vi "Test Process within Nested App Log When Logger Set for Intermediate App.vi"(8 "error in (no error)":errorcluster, 11 "Test Case In":refnum<class "Logger Test.lvclass">) -> (0 "error out":errorcluster, 3 "Test Case Out":refnum<class "Logger Test.lvclass">)   [LabVIEW 2020, in "Logger Test.lvclass"]
uses:
  Logger Test.lvclass
  Logger Test.lvclass/Logger Test.ctl
  source/Framework Test Suite/Mock Log Handler/Mock Log Handler.lvclass
  source/Framework/Process/Process.lvclass
  source/Framework/Application/Application.lvclass
  source/Framework Test Suite/Mock Process/Mock Process.lvclass
  source/Framework Test Suite/Support/Test Support.lvlib
  source/Framework/Logging/Logging.lvclass
  9c4a66fc-af29-4a58-8a71-606aefca4567.vi
  C:/Git/astemes-triarc-framework/source/Framework/Process/Process.lvclass
  C:/Git/astemes-triarc-framework/source/Framework/Base/Base.lvclass
  C:/Git/astemes-triarc-framework/source/Framework/Error Handler Interface/Error Handler Interface.lvclass
  C:/Git/astemes-triarc-framework/source/Framework/Logging/Logging.lvclass
  C:/Git/astemes-triarc-framework/source/Framework/Application/Application.lvclass
  C:/Git/astemes-triarc-framework/source/Framework/Async Handler/Async Handler.lvclass
  C:/Git/astemes-triarc-framework/source/Framework Test Suite/Mock Log Handler/Mock Log Handler.lvclass
  C:/Git/astemes-triarc-framework/source/Framework/Configuration File/Configuration File.lvclass
  C:/Git/astemes-triarc-framework/source/Framework/Configuration/Configuration.lvclass
  C:/Git/astemes-triarc-framework/source/Framework Test Suite/Mock Process/Mock Process.lvclass
  C:/Git/astemes-triarc-framework/source/Framework/Helper Loop/Helper Loop.lvclass
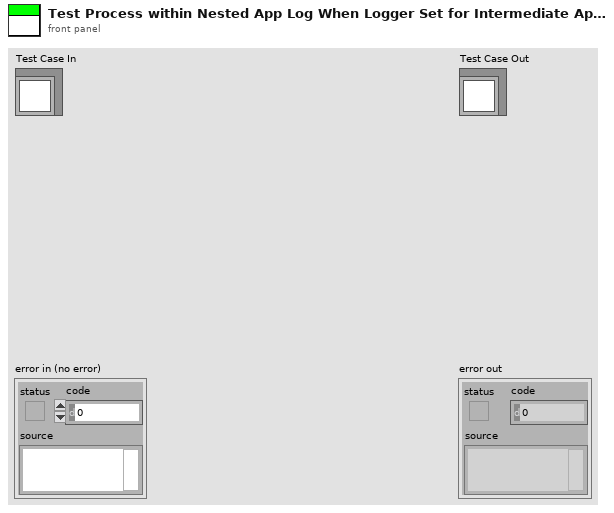
[diagram p1: front panel]
types:
  T1 = typedef "Mock Log Handler.lvclass/Log Entry.ctl" = cluster{"Level":string, "Source":string, "Message":string}
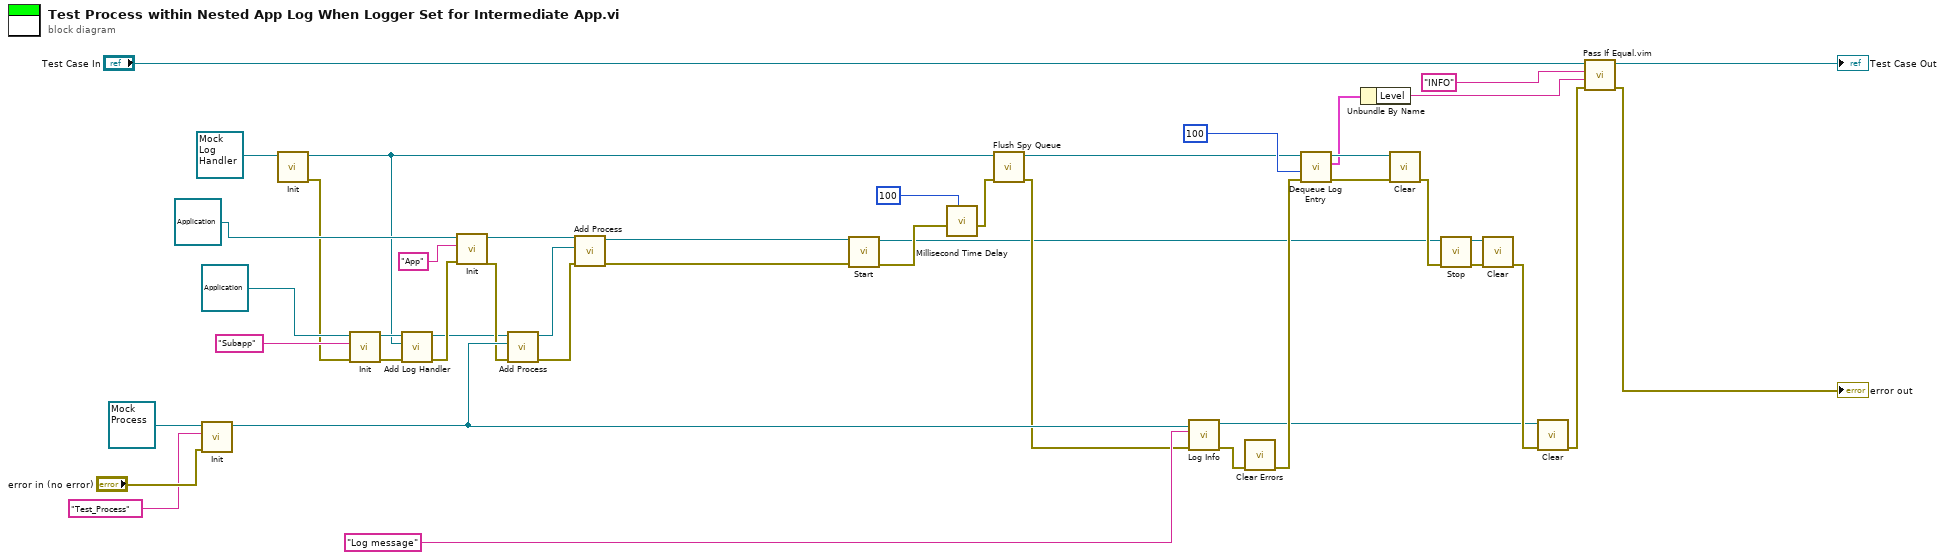
[diagram p0: block diagram]
diagram:
  n1 = call-dynamic "Init.vi"("error in (no error)"="error in (no error)", "Name"="Test_Process", "Mock Process In"=refnum<class "Mock Process.lvclass"> refnum) -> ("Mock Process Out"=w18:refnum<class "Mock Process.lvclass">)  [unwired: 7 in, 1 out]
  n2 = call-dynamic "Init.vi"("Mock Log Handler In"=refnum<class "Mock Log Handler.lvclass"> refnum ("Mock Log Handler.lvclass")) -> ("error out"=w6:errorcluster, "Mock Log Handler Out"=w1:refnum<class "Mock Log Handler.lvclass">)  [unwired: 9 in]
  n3 = call-dynamic "Init.vi"("error in (no error)"=w6, "Name"="Subapp", "Process In"=refnum<class "Application.lvclass"> refnum ("Application.lvclass")) -> ("error out"=w5:errorcluster, "Process Out"=w3:refnum<class "Application.lvclass">)  [unwired: 7 in]
  n4 = call "Add Log Handler.vi"("error in (no error)"=w5, "Log Handler"=w1, "Process In"=w3) -> ("error out"=w4:errorcluster, "Process Out"=w2:refnum<class "Application.lvclass">)  [unwired: 7 in]
  n5 = call-dynamic "Init.vi"("error in (no error)"=w4, "Name"="App", "Process In"=refnum<class "Application.lvclass"> refnum ("Application.lvclass")) -> ("error out"=w13:errorcluster, "Process Out"=w15:refnum<class "Application.lvclass">)  [unwired: 7 in]
  n6 = call "Add Process.vi"("error in (no error)"=w13, "Process"=w18, "Application In"=w2) -> ("error out"=w12:errorcluster, "Application Out"=w14:refnum<class "Application.lvclass">)  [unwired: 7 in]
  n7 = call "Add Process.vi"("error in (no error)"=w12, "Process"=w14, "Application In"=w15) -> ("error out"=w11:errorcluster, "Application Out"=w9:refnum<class "Application.lvclass">)  [unwired: 7 in]
  n8 = call "Start.vi"("error in (no error)"=w11, "Process In"=w9) -> ("error out"=w10:errorcluster, "Process Out"=w8:refnum<class "Application.lvclass">)  [unwired: 7 in, 1 out]
  n9 = call "Millisecond Time Delay.vi"("milliseconds to wait"=u32 100, "error in (no error)"=w10) -> ("error out"=w20:errorcluster)  [unwired: 7 in]
  n10 = call "Flush Spy Queue.vi"("error in (no error)"=w20, "Mock Log Handler in"=w1) -> ("error out"=w17:errorcluster, "Mock Log Handler out"=w21:refnum<class "Mock Log Handler.lvclass">)  [unwired: 7 in, 1 out]
  n11 = call "Log Info.vi"("error in (no error)"=w17, "Message"="Log message", "Logging In"=w18) -> ("error out"=w31:errorcluster, "Logging Out"=w22:refnum<class "Mock Process.lvclass">)  [unwired: 7 in]
  n12 = call <vilib>:"Clear Errors.vi"("error in (no error)"=w31) -> ("error out"=w30:errorcluster)  [unwired: 5 in, 1 out]
  n13 = call "Dequeue Log Entry.vi"("error in (no error)"=w30, "timeout in ms (-1)"=100, "Mock Log Handler in"=w21) -> ("error out"=w40:errorcluster, "Entry"=w37:T1, "Mock Log Handler out"=w41:refnum<class "Mock Log Handler.lvclass">)  [unwired: 5 in, 1 out]
  n14 = Unbundle By Name(w37) -> ("Level"=w36:string)
  n15 = call-dynamic "Clear.vi"("error in (no error)"=w40, "Mock Log Handler In"=w41) -> ("error out"=w38:errorcluster)  [unwired: 9 in]
  n16 = call "Stop.vi"("error in (no error)"=w38, "Process In"=w8) -> ("error out"=w24:errorcluster, "Process Out"=w23:refnum<class "Application.lvclass">)  [unwired: 7 in, 1 out]
  n17 = call-dynamic "Clear.vi"("error in (no error)"=w24, "Application In"=w23) -> ("error out"=w43:errorcluster)  [unwired: 9 in]
  n18 = call-dynamic "Clear.vi"("error in (no error)"=w43, "Mock Process In"=w22) -> ("error out"=w33:errorcluster)  [unwired: 9 in]
  n19 = call "Pass If Equal.vim"("error in (no error)"=w33, "Actual"=w36, "Expected"="INFO", "LUnit Test Case In"="Test Case In") -> ("error out"=→"error out":errorcluster, "LUnit Test Case Out"=→"Test Case Out":refnum<class "Logger Test.lvclass">)  [unwired: 6 in]
